vi "Dynamic Component UI.vi"() -> ()   [LabVIEW 2017]
uses:
  DSF Core.lvlibp/Classes/Component User Interface/UI Type.ctl
  DSF Core.lvlibp/Typedefs/DSF Settings Info.ctl
  DSF Core.lvlibp/Typedefs/DSF Version Info.ctl
  DSF Core.lvlibp/Classes/Configuration/Configuration.lvclass
  DSF Core.lvlibp/Classes/User Interface/Plugin/Component Settings Editor.lvclass
  DSF Core.lvlibp/Classes/User Interface Handler/User Interface Handler.lvclass
  DSF Core.lvlibp/Classes/Component Loader/Component Loader.lvclass
  DSF Core.lvlibp/Classes/Component User Interface/Component User Interfaces.lvclass
  DSF Core.lvlibp/Classes/Component/Component.lvclass
  DSF Core.lvlibp/Classes/User Interface/User Interface.lvclass
  DSF Core.lvlibp/Classes/Component Configuration/Component Configurations.lvclass
  DSF Core.lvlibp
  C:/Git/DSF/VeriStand/Data Sharing Custom Device/Source/DSF Core.lvlibp/Classes/User Interface/User Interface.lvclass
panel:
  out "settings":cluster{"key":string, "value":string}[](array[cluster])
  in  "component names":string[](array[string])
  in  "components directory":path
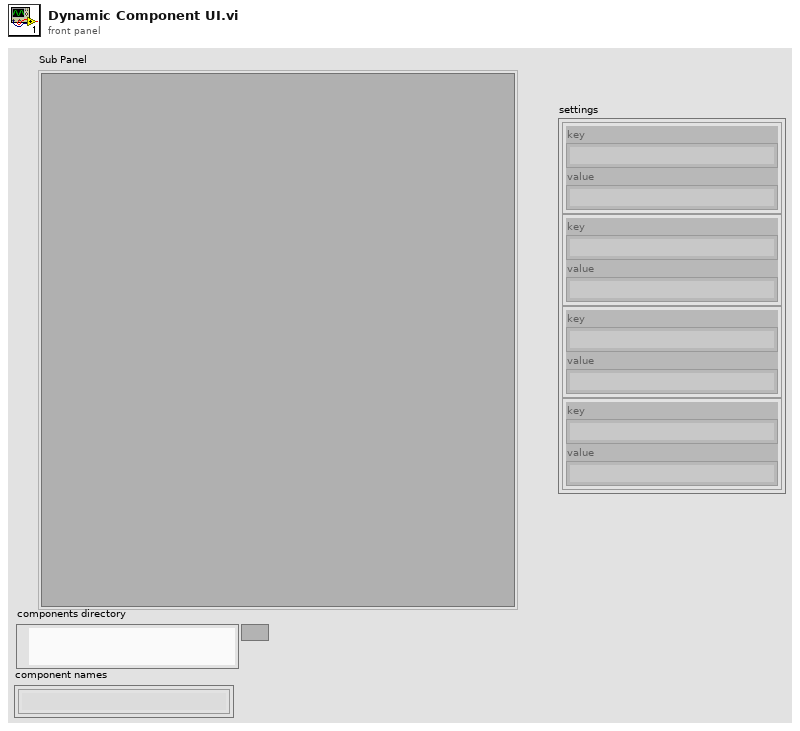
[diagram p1: front panel]
types:
  T1 = typedef "DSF Core.lvlibp/DSF Settings Info.ctl" = cluster{"component":string, "version":T2, "values":cluster{"key":string, "value":string}[]}
  T2 = typedef "DSF Core.lvlibp/DSF Version Info.ctl" = cluster{"major":u32, "minor":u32, "fix":u32, "build":string}
  T3 = typedef "DSF Core.lvlibp/Component User Interfaces.lvclass/UI Type.ctl" = enum16{"Plugin", "Thread", "Rx Group", "Tx Group", "Rx Transfer", "Tx Transfer", "Rx Channel", "Tx Channel"}
  T4 = typedef "DSF Core.lvlibp/User Interface Handler.lvclass/User Interface Ref.ctl" = refnum<vi>
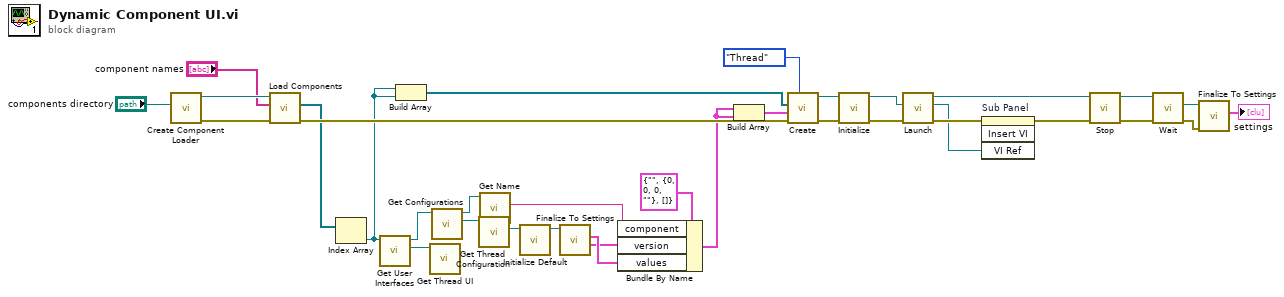
[diagram p0: block diagram]
diagram:
  n1 = call "Create Component Loader.vi"("components directory (default)"="components directory") -> ("error out"=w26:errorcluster, "Component Loader out"=w29:refnum<class "Component Loader.lvclass">)  [unwired: 9 in]
  n2 = call "Load Components.vi"("error in (no error)"=w26, "component names"="component names", "Component Loader in"=w29) -> ("error out"=w28:errorcluster, "Components"=w22:refnum<class "Component.lvclass">[])  [unwired: 6 in, 1 out]
  n3 = Index Array(array=w22) -> (element=w6:refnum<class "Component.lvclass">)  [unwired: 1 in]
  n4 = call "Get User Interfaces.vi"("Component in"=w6) -> ("User Interfaces"=w21:refnum<class "Component User Interfaces.lvclass">, "Component out"=w14:refnum<class "Component.lvclass">)  [unwired: 9 in]
  n5 = Build Array(w6, w6) -> (w4:refnum<class "Component.lvclass">[])
  n6 = call "Get Thread UI.vi"("Component UI in"=w21) -> ()  [unwired: 8 in, 3 out]
  n7 = call "Get Configurations.vi"("Component in"=w14) -> ("Configurations"=w13:refnum<class "Component Configurations.lvclass">, "Component out"=w11:refnum<class "Component.lvclass">)  [unwired: 9 in]
  n8 = call "Get Thread Configuration.vi"("Component Configuration in"=w13) -> ("Thread Configuration"=w3:refnum<class "Configuration.lvclass">)  [unwired: 8 in, 2 out]
  n9 = call "Get Name.vi"("Component in"=w11) -> ("name"=w8:string)  [unwired: 9 in, 1 out]
  n10 = call-dynamic "Initialize Default.vi"("Configuration in"=w3) -> ("Configuration out"=w2:refnum<class "Configuration.lvclass">)  [unwired: 9 in, 1 out]
  n11 = call-dynamic "Finalize To Settings.vi"("Configuration in"=w2) -> ("settings version"=w9:T2, "settings"=w10:cluster{"key":string, "value":string}[])  [unwired: 7 in, 2 out]
  n12 = Bundle By Name(cluster=T1 {"component"="", "version"={"major"=0, "minor"=0, "fix"=0, "build"=""}, "values"=[]} ("component settings"), "component"=w8, "version"=w9, "values"=w10) -> (w5:T1)
  n13 = Build Array(w5, w5) -> (w7:T1[])
  n14 = call "Create.vi"("user interface type"=UI_Type."Thread", "error in (no error)"=w28, "component settings"=w7, "Components"=w4) -> ("error out"=w17:errorcluster, "Component Settings Editor out"=w18:refnum<class "Component Settings Editor.lvclass">)  [unwired: 6 in]
  n15 = call-dynamic "Initialize.vi"("error in (no error)"=w17, "Component Settings Editor in"=w18) -> ("error out"=w30:errorcluster, "Component Settings Editor out"=w1:refnum<class "Component Settings Editor.lvclass">)  [unwired: 8 in]
  n16 = call "Launch.vi"("error in (no error)"=w30, "User Interface"=w1) -> ("error out"=w24:errorcluster, "active vi"=w23:T4, "User Interface Handler out"=w34:refnum<class "User Interface Handler.lvclass">)  [unwired: 7 in]
  n17 = invoke on="Sub Panel" class="SubPnl" method="Insert VI"(error in=w24, "VI Ref"=w23) -> (error out=w31:errorcluster)  [unwired: 2 in, 3 out]
  n18 = call "Stop.vi"("error in (no error)"=w31, "User Interface Handler in"=w34) -> ("error out"=w32:errorcluster, "User Interface Handler out"=w33:refnum<class "User Interface Handler.lvclass">)  [unwired: 8 in]
  n19 = call "Wait.vi"("error in (no error)"=w32, "User Interface Handler in"=w33) -> ("error out"=w15:errorcluster, "User Interface"=w20:refnum<class "User Interface.lvclass">)  [unwired: 7 in, 1 out]
  n20 = call "Finalize To Settings.vi"("error in (no error)"=w15, "User Interface in"=w20) -> ("settings"=→"settings":cluster{"key":string, "value":string}[])  [unwired: 6 in, 3 out]
